vi "Create Comm Parms.vi"() -> (0 "error out":errorcluster, 1 "VISA resource name out":refnum<visa-resource-name>)   [LabVIEW 2012]
uses:
  Type Defs/Comm Settings.ctl
panel:
  in  "Port":refnum<visa-resource-name>
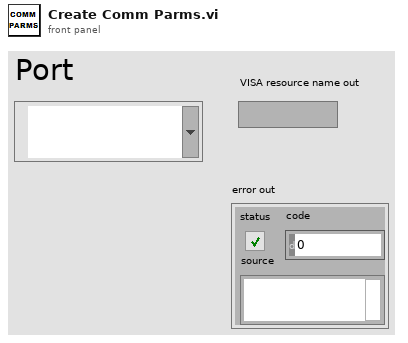
[diagram p1: front panel]
types:
  T1 = typedef "Comm Settings.ctl" = cluster{"Port":refnum<visa-resource-name>, "Baud Rate":u32, "Data Bits":u16, "Parity":u16, "Stop Bits":u16, "Flow Control":u16}
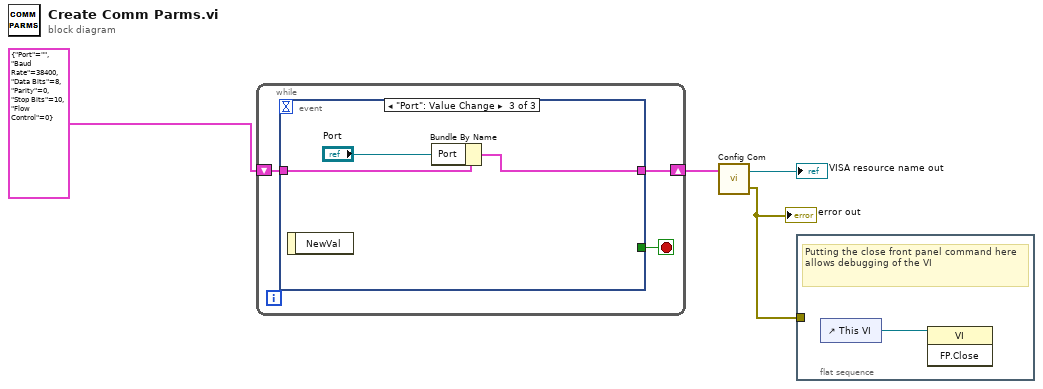
[diagram p0: block diagram]
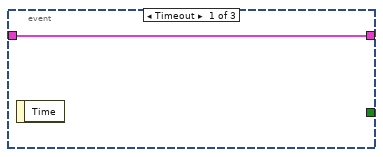
[diagram p2: hidden frame]
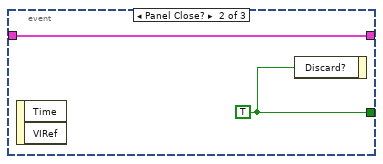
[diagram p3: hidden frame]
diagram:
  n1 = while {
    shift-right: [w6] -> w4
    shift-left: T1 {"Port"="", "Baud Rate"=38400, "Data Bits"=8, "Parity"=0, "Stop Bits"=10, "Flow Control"=0} ("Com Parms") -> [w7]
    stop <- w5 stop-if-true
    n2 = event shown="[2] \"Port\": Value Change" {
      selector: _ -> [_ _ _]
      dyn-events: _ -> [_ _ _]
      timeout: _ -> [_ _ _]
      tunnel: [w8 w10 w11] -> w6
      tunnel: w7 -> [w8 w10 w13]
      tunnel: [_ w9 _] -> w5
      event Timeout {
        n3 = event-data() -> ()  [unwired: 1 in, 1 out]
      }
      event Panel Close? {
        w9 = TRUE
        n4 = event-data() -> ()  [unwired: 1 in, 2 out]
        n5 = event-data("Discard?"=w9) -> ()  [unwired: 1 in, 1 out]
      }
      event "Port": Value Change {
        n6 = event-data() -> ()  [unwired: 1 in, 1 out]
        n7 = Bundle By Name(cluster=w13, "Port"="Port") -> (w11:T1)
      }
    }
  }
  n8 = call "Config Com.vi"("Com Parms"=w4) -> ("error out"=w2:errorcluster, "VISA resource name out"=→"VISA resource name out":refnum<visa-resource-name>)  [unwired: 1 in]
  "error out" <- w2
  n9 = flat-sequence {
    tunnel: w2 -> [_]
    frame #0 {
      # "Putting the close front panel command here allows debugging of the VI"
      n10 = control-ref of="This VI"() -> (w14:refnum<vi>)
      n11 = invoke class="VI" method="FP.Close"(reference=w14) -> ()  [unwired: 2 in, 3 out]
    }
  }
